vi "raddrizzatore_bipolare.vi"(2 "waveform":waveform(dbl)) -> (0 "output waveform":waveform(dbl))   [LabVIEW 2009]
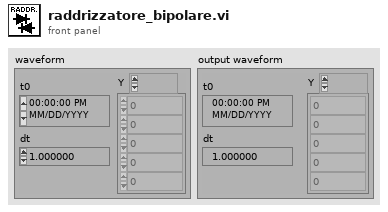
[diagram p1: front panel]
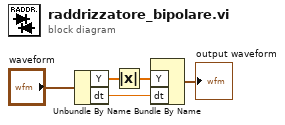
[diagram p0: block diagram]
diagram:
  n1 = Unbundle By Name("waveform") -> ("Y"=w4:dbl[], "dt"=w2:dbl)
  n2 = Absolute Value(x=w4) -> (abs(x)=w3:dbl[])
  n3 = Bundle By Name("Y"=w3, "dt"=w2) -> (→"output waveform":waveform(dbl))  [unwired: 1 in]
